vi "Mean (DBL).vi"(0 "X":dbl[](array[numeric]) format="%0.2f") -> (1 "mean":dbl format="%0.2f", 2 "error":i32)   [LabVIEW 2013, in "NI_AALBase.lvlib"]
doc: "Computes the <B>mean</B> of the values in the input sequence <B>X</B>. You must manually select the polymorphic instance you want to use."
uses:
  NI_AALBase.lvlib
  lvanlys.dll
panel:
  # "Mean"
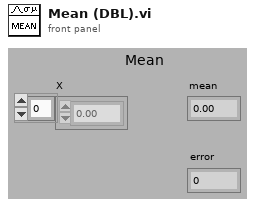
[diagram p1: front panel]
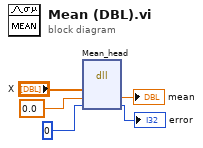
[diagram p0: block diagram]
diagram:
  n1 = dll-call lib="C:/Program Files (x86)/National Instruments/LabVIEW 2013/resource/lvanlys.*" fn="Mean_head"("X"="X", "output param"=0.0, "output param"=0) -> ("output param"=→"mean":dbl, "output param"=→"error":i32)  [unwired: 5 in, 2 out]
